vi "GetText.vi"(8 "error in":errorcluster, 11 "node in":refnum<class "Pages.lvclass">) -> (0 "error out":errorcluster, 1 "additional text":string, 2 "text":string, 3 "node out":refnum<class "Pages.lvclass">, 4 "glyph":string)   [LabVIEW 2015, in "Pages.lvclass"]
doc: "Returns the text representation of the node used for the tree control."
uses:
  Pages.lvclass
  Pages.lvclass/Pages.ctl
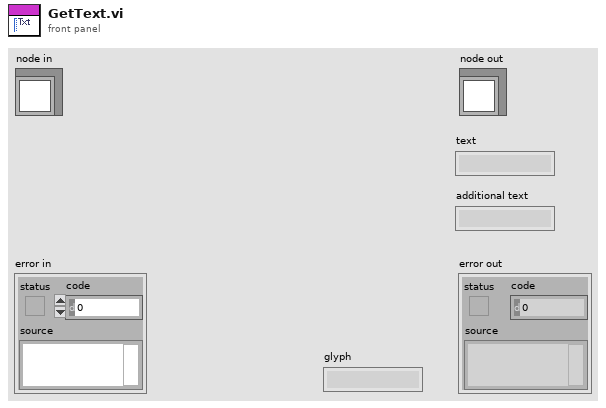
[diagram p1: front panel]
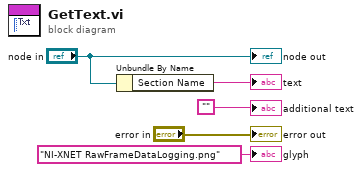
[diagram p0: block diagram]
diagram:
  n1 = Unbundle By Name("node in") -> ("Section Name"=→"text":string)
  "error out" <- "error in"
  "node out" <- "node in"
  "additional text" <- ""
  "glyph" <- "NI-XNET RawFrameDataLogging.png" ("glyph")
